vi "Transfer.Get Size.vi"(11 "Transfer in":refnum<class "Transfer.lvclass">) -> (2 "size":u64, 3 "Transfer out":refnum<class "Transfer.lvclass">)   [LabVIEW 2017, in "DSF.Engine.lvlib" / "Transfer.lvclass"]
uses:
  Transfer.lvclass
  Transfer.lvclass/Transfer.ctl
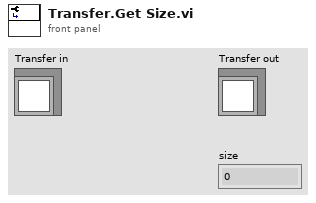
[diagram p1: front panel]
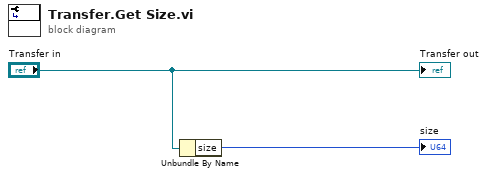
[diagram p0: block diagram]
diagram:
  n1 = Unbundle By Name("Transfer in") -> ("size"=→"size":u64)
  "Transfer out" <- "Transfer in"
